vi "Open Me.vi"   [LabVIEW 2016]
uses:
  <userlib>/LevyLab/Levylab Instruments/Instrument Types/Cryostat/Instrument.Cryostat.lvclass
  Control Experiment/Control Experiment.lvclass
  SweepControl/SweepControl.lvclass
  Transport/Transport.lvclass
panel:
  # "Open the block diagram"
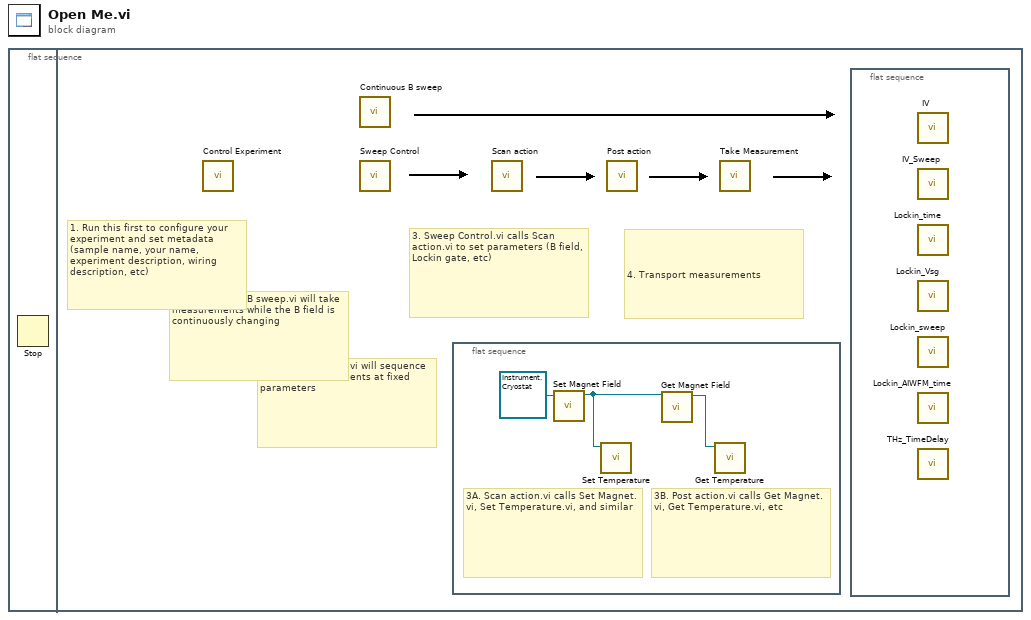
[diagram p0: block diagram]
diagram:
  n1 = flat-sequence {
    frame #0 {
      n2 = Stop() -> ()  [unwired: 1 in]
    }
    frame #1 {
      # "2A. Sweep Control.vi will sequence a set of measurements at fixed parameters"
      # "2B. Continuous B sweep.vi will take measurements while the B field is continuously changing"
      # "4. Transport measurements"
      # "3. Sweep Control.vi calls Scan action.vi to set parameters (B field, Lockin gate, etc)"
      # "1. Run this first to configure your experiment and set metadata (sample name, your name, experiment description, wiring description, etc)"
      n3 = call "Control Experiment.vi"() -> ()  [unwired: 11 in, 1 out]
      n4 = call "Continuous B sweep.vi"() -> ()  [unwired: 11 in, 1 out]
      n5 = call "Sweep Control.vi"() -> ()  [unwired: 11 in, 1 out]
      n6 = flat-sequence {
        frame #0 {
          # "3B. Post action.vi calls Get Magnet.vi, Get Temperature.vi, etc"
          # "3A. Scan action.vi calls Set Magnet.vi, Set Temperature.vi, and similar"
          n7 = call-dynamic "Set Magnet Field.vi"("Instrument.Cryostat in"=refnum<class "Instrument.Cryostat.lvclass"> refnum) -> ("Instrument.Cryostat out"=w3:refnum<class "Instrument.Cryostat.lvclass">)  [unwired: 9 in, 1 out]
          n8 = call-dynamic "Set Temperature.vi"("Instrument.Cryostat in"=w3) -> ()  [unwired: 9 in, 2 out]
          n9 = call-dynamic "Get Magnet Field.vi"("Instrument.Cryostat in"=w3) -> ("Instrument.Cryostat out"=w1:refnum<class "Instrument.Cryostat.lvclass">)  [unwired: 6 in, 4 out]
          n10 = call-dynamic "Get Temperature.vi"("Instrument.Cryostat in"=w1) -> ()  [unwired: 6 in, 5 out]
        }
      }
      n11 = call "Scan action.vi"() -> ()  [unwired: 9 in, 3 out]
      n12 = call "Post action.vi"() -> ()  [unwired: 10 in, 2 out]
      n13 = call "Take Measurement.vi"() -> ()  [unwired: 8 in, 4 out]
      n14 = flat-sequence {
        frame #0 {
          n15 = call "IV.vi"() -> ()  [unwired: 10 in, 2 out]
          n16 = call "IV_Sweep.vi"() -> ()  [unwired: 10 in, 2 out]
          n17 = call "Lockin_time.vi"() -> ()  [unwired: 10 in, 2 out]
          n18 = call "Lockin_Vsg.vi"() -> ()  [unwired: 10 in, 2 out]
          n19 = call "Lockin_sweep.vi"() -> ()  [unwired: 10 in, 2 out]
          n20 = call "Lockin_AIWFM_time.vi"() -> ()  [unwired: 10 in, 2 out]
          n21 = call "THz_TimeDelay.vi"() -> ()  [unwired: 10 in, 2 out]
        }
      }
    }
  }
